vi "Create NXT Timer Index.vi"(1 "Timer (Timer 1)":T1 items=["Timer 1", "Timer 2", "Timer 3"]) -> (0 "Branched Timer Index":T2)   [LabVIEW 2010, in "timerExts.lvlib"]
uses:
  timerExts.lvlib
  Branched Timer.ctl
  <vilib>/NXT/Block Support/NXT_TimerIndex.ctl
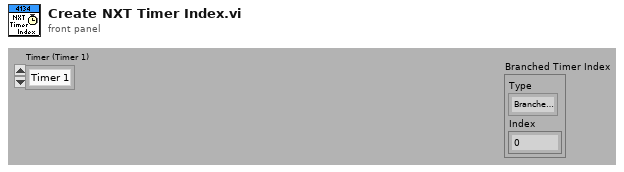
[diagram p1: front panel]
types:
  T1 = typedef "NXT_TimerIndex.ctl" = u8
  T2 = typedef "timerExts.lvlib/Branched Timer.ctl" = cluster{"Type":enum8{"Branched Timer", "NXT Timer"}, "Index":u16}
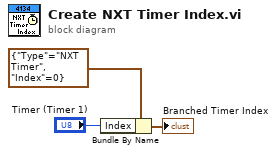
[diagram p0: block diagram]
diagram:
  n1 = Bundle By Name(cluster=T2 {"Type"=enum."NXT Timer", "Index"=0} ("Branched Timer Index 2"), "Index"="Timer (Timer 1)") -> (→"Branched Timer Index":T2)
